vi "Write Log Header.vi"(8 "error in (no error)":errorcluster, 11 "Model in":refnum<class "Model.lvclass">) -> (0 "error out":errorcluster, 3 "Model out":refnum<class "Model.lvclass">)   [LabVIEW 2016, in "Model.lvclass"]
uses:
  Model.lvclass
  Model.lvclass/Model.ctl
  Test Log/Test Log/OperationsLog.lvclass
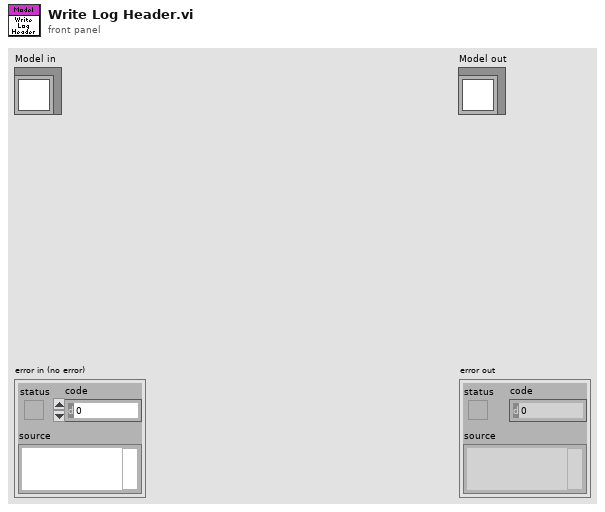
[diagram p1: front panel]
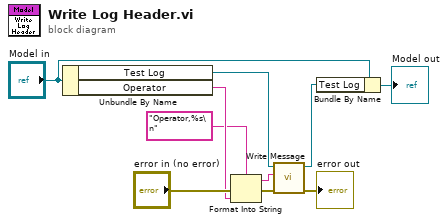
[diagram p0: block diagram]
diagram:
  n1 = Unbundle By Name("Model in") -> ("Test Log"=w9:refnum<class "OperationsLog.lvclass">, "Operator"=w2:string)
  n2 = Format Into String(format string="Operator,%s\n", error in="error in (no error)", w2) -> (resulting string=w10:string, error out=w6:errorcluster)  [unwired: 1 in]
  n3 = call-dynamic "Write Message.vi"("error in (no error)"=w6, "Message"=w10, "Test Log in"=w9) -> ("error out"=→"error out":errorcluster, "Test Log out"=w8:refnum<class "OperationsLog.lvclass">)  [unwired: 7 in]
  n4 = Bundle By Name(cluster="Model in", "Test Log"=w8) -> (→"Model out":refnum<class "Model.lvclass">)
